vi "ChangeYourDisk.vi"() -> ()   [LabVIEW 2014]
panel:
  in  "Stop Button":bool
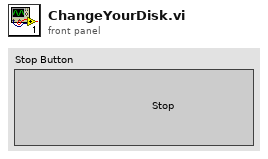
[diagram p1: front panel]
types:
  T1 = enum16{"open", "replace", "create", "open or create", "replace or create", "replace or create with confirmation"}
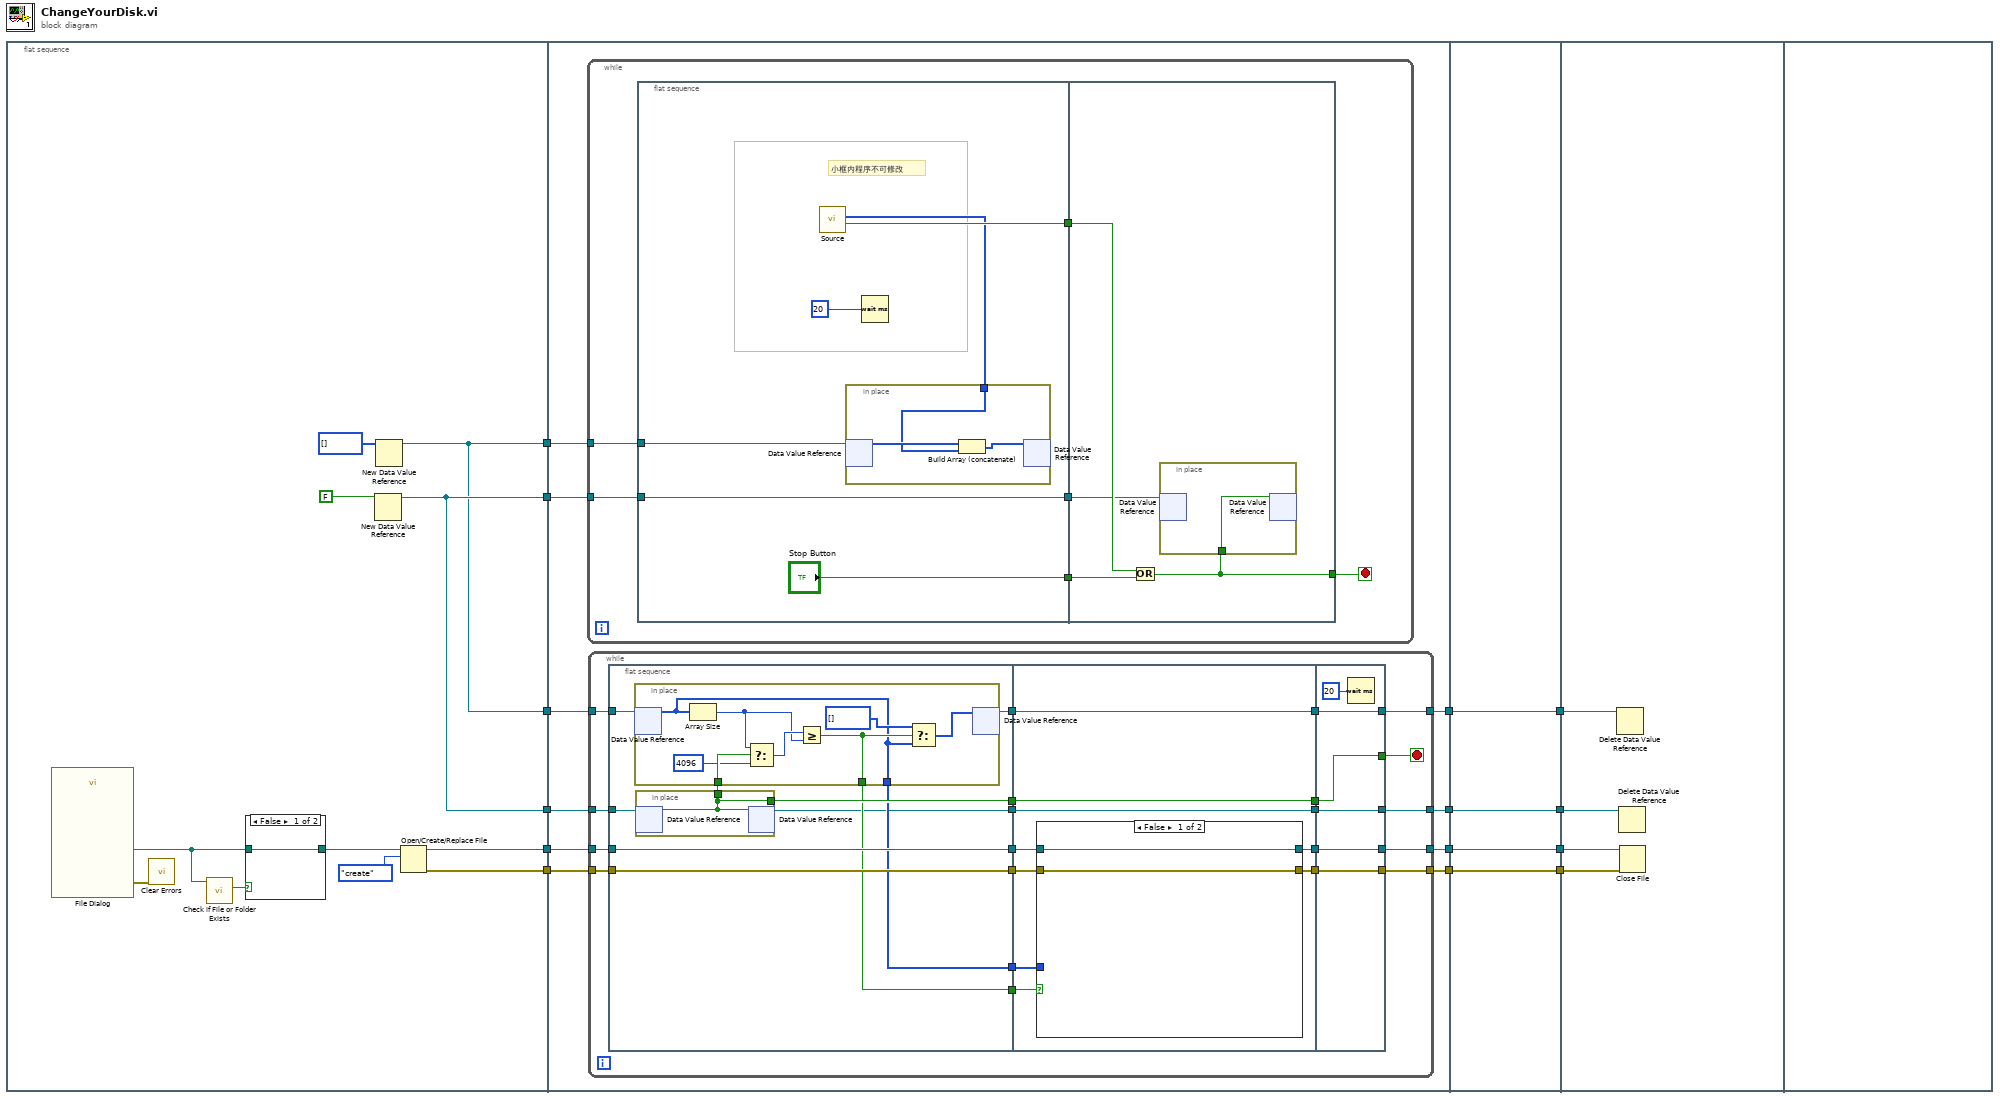
[diagram p0: block diagram]
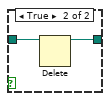
[diagram p2: hidden frame]
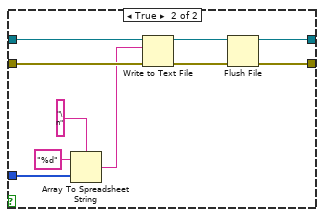
[diagram p3: hidden frame]
diagram:
  n1 = flat-sequence {
    tunnel: [w19] -> w14
    tunnel: [w18] -> w13
    tunnel: [w15] -> w12
    tunnel: [w16] -> w10
    tunnel: [w16] -> w2
    tunnel: [w15] -> w1
    tunnel: w14 -> [w38]
    tunnel: w13 -> [w37]
    tunnel: w12 -> [w36]
    tunnel: [w35] -> w11
    tunnel: w10 -> [w34]
    tunnel: [w33] -> w8
    tunnel: [w32] -> w7
    tunnel: [w31] -> w4
    tunnel: w2 -> [w30]
    tunnel: w1 -> [w29]
    tunnel: w11 -> [w127]
    tunnel: [w129] -> w9
    tunnel: w8 -> [w129]
    tunnel: w7 -> [w128]
    tunnel: [w128] -> w6
    tunnel: [w127] -> w5
    tunnel: w4 -> [w126]
    tunnel: [w126] -> w3
    tunnel: w9 -> [w133]
    tunnel: w6 -> [w132]
    tunnel: w5 -> [w131]
    tunnel: w3 -> [w130]
    frame #0 {
      n2 = call "File Dialog"() -> ("selected path"=w22:path, "error out"=w24:errorcluster)  [unwired: 12 in, 2 out]
      n3 = call <vilib>:"Clear Errors.vi"("error in (no error)"=w24) -> ()  [unwired: 5 in, 2 out]
      n4 = call <vilib>:"Check if File or Folder Exists.vi"("path"=w22) -> ("file or folder exists?"=w23:bool)  [unwired: 8 in, 2 out]
      n5 = case shown="False" w23 {
        tunnel: w22 -> [w26 w28]
        tunnel: [w26 w27] -> w21
        frame False {
        }
        frame True {
          n6 = Delete(path (use dialog)=w28) -> (deleted path=w27:path)  [unwired: 4 in, 2 out]
        }
      }
      n7 = New Data Value Reference(data value=FALSE) -> (data value reference=w16:refnum<data-value>)  [unwired: 1 in, 1 out]
      n8 = New Data Value Reference(data value=i16[] []) -> (data value reference=w15:refnum<data-value>)  [unwired: 1 in, 1 out]
      n9 = Open/Create/Replace File(file path (use dialog)=w21, operation (0:open)=T1."create") -> (refnum out=w19:refnum<file>, error out=w18:errorcluster)  [unwired: 4 in, 1 out]
    }
    frame #1 {
      n10 = while {
        tunnel: w30 -> [w107]
        tunnel: w29 -> [w106]
        stop <- w110 stop-if-true
        n11 = flat-sequence {
          tunnel: ["Stop Button"] -> w111
          tunnel: [w116] -> w109
          tunnel: [w114] -> w108
          tunnel: w107 -> [w114]
          tunnel: w106 -> [w113]
          tunnel: w111 -> [w124]
          tunnel: [w121] -> w110
          tunnel: w109 -> [w123]
          tunnel: w108 -> [w122]
          frame #0 {
            # "小框内程序不可修改"
            n12 = call "Source.vi"() -> ("Terminate?"=w116:bool, "output"=w112:i16[])  [unwired: 2 in]
            n13 = in-place {
              in-place-border: w112 -> [w119]
              n14 = in-place-dvr #1(w113) -> (w120:i16[])  [unwired: 1 out]
              n15 = Build Array (concatenate)(w120, w119) -> (w118:i16[])
              n16 = in-place-dvr #1(w118) -> ()  [unwired: 2 out]
            }
            n17 = Wait (ms)(milliseconds to wait=u32 20) -> ()  [unwired: 1 out]
          }
          frame #1 {
            n18 = Or(x=w123, y=w124) -> (x .or. y?=w121:bool)
            n19 = in-place {
              in-place-border: w121 -> [w125]
              n20 = in-place-dvr #2(w122) -> ()  [unwired: 2 out]
              n21 = in-place-dvr #2(w125) -> ()  [unwired: 2 out]
            }
          }
        }
      }
      n22 = while {
        tunnel: w38 -> [w59]
        tunnel: w37 -> [w58]
        tunnel: w36 -> [w57]
        tunnel: [w54] -> w35
        tunnel: w34 -> [w53]
        tunnel: [w44] -> w33
        tunnel: [w42] -> w32
        tunnel: [w39] -> w31
        stop <- w50 stop-if-true
        n23 = flat-sequence {
          tunnel: w59 -> [w64]
          tunnel: w58 -> [w63]
          tunnel: w57 -> [w69]
          tunnel: [w68] -> w55
          tunnel: w53 -> [w67]
          tunnel: [w65] -> w52
          tunnel: [w64] -> w49
          tunnel: [w63] -> w48
          tunnel: [w62] -> w47
          tunnel: [w61] -> w46
          tunnel: [w60] -> w41
          tunnel: [w87] -> w56
          tunnel: w55 -> [w87]
          tunnel: w52 -> [w86]
          tunnel: [w86] -> w51
          tunnel: w49 -> [w85]
          tunnel: w48 -> [w84]
          tunnel: w47 -> [w83]
          tunnel: w46 -> [w82]
          tunnel: [w81] -> w45
          tunnel: [w80] -> w43
          tunnel: w41 -> [w79]
          tunnel: [w79] -> w40
          tunnel: [w104] -> w54
          tunnel: w56 -> [w104]
          tunnel: w51 -> [w103]
          tunnel: [w103] -> w50
          tunnel: w45 -> [w102]
          tunnel: [w102] -> w44
          tunnel: w43 -> [w101]
          tunnel: [w101] -> w42
          tunnel: w40 -> [w100]
          tunnel: [w100] -> w39
          frame #0 {
            n24 = in-place {
              in-place-border: [w70] -> w66
              in-place-border: [w70] -> w65
              n25 = in-place-dvr #3(w67) -> (w70:bool)  [unwired: 1 out]
              n26 = in-place-dvr #3(w70) -> (w60:refnum<data-value>)  [unwired: 1 out]
            }
            n27 = in-place {
              in-place-border: w66 -> [w78]
              in-place-border: [w72] -> w62
              in-place-border: [w71] -> w61
              n28 = in-place-dvr #4(w69) -> (w71:i16[])  [unwired: 1 out]
              n29 = Array Size(array=w71) -> (size(s)=w75:i32)
              n30 = Select(t=w75, s=w78, f=i16 4096 ("y")) -> (s? t:f=w76:i32)
              n31 = Greater Or Equal?(x=w76, y=w75) -> (x >= y?=w72:bool)
              n32 = Select(t=i16[] [] ("f"), s=w72, f=w71) -> (s? t:f=w74:i16[])
              n33 = in-place-dvr #4(w74) -> (w68:refnum<data-value>)  [unwired: 1 out]
            }
          }
          frame #1 {
            n34 = case shown="False" w83 {
              tunnel: w85 -> [w89 w96]
              tunnel: w84 -> [w88 w95]
              tunnel: w82 -> [_ w99]
              tunnel: [w89 w91] -> w81
              tunnel: [w88 w90] -> w80
              frame False {
              }
              frame True {
                n35 = Array To Spreadsheet String(delimiter (Tab)="\n", array=w99, 3:"%d" ("format string")) -> (spreadsheet string=w94:string)
                n36 = Write to Text File(file (use dialog)=w96, text=w94, error in=w95) -> (refnum out=w93:refnum<file>, error out=w92:errorcluster)  [unwired: 1 in, 1 out]
                n37 = Flush File(refnum=w93, error in=w92) -> (refnum out=w91:refnum<file>, error out=w90:errorcluster)
              }
            }
          }
          frame #2 {
            n38 = Wait (ms)(milliseconds to wait=u32 20) -> ()  [unwired: 1 out]
          }
        }
      }
    }
    frame #2 {
    }
    frame #3 {
      n39 = Delete Data Value Reference(data value reference=w131) -> ()  [unwired: 1 in, 2 out]
      n40 = Delete Data Value Reference(data value reference=w130) -> ()  [unwired: 1 in, 2 out]
      n41 = Close File(refnum=w133, error in=w132) -> ()  [unwired: 2 out]
    }
    frame #4 {
    }
  }
